vi "CCD Exposure Time Control.vi"(8 "error in (no error)":errorcluster, 11 "CCD in":refnum<class "CCD.lvclass">) -> (0 "error out":errorcluster, 3 "CCD out":refnum<class "CCD.lvclass">)   [LabVIEW 2020, in "Examples.lvlib"]
doc: "Example on how to use the timer resolution to to achieve a exposure time in mili seconds."
uses:
  Examples.lvlib
  Classes/CCD/CCD.lvclass
panel:
  out "time [ms] or [us]":i32
  out "resolutionToken":i32
  # "See Block Diagram\nfor explanation"
  # "Connector Pane"
  # "Locals"
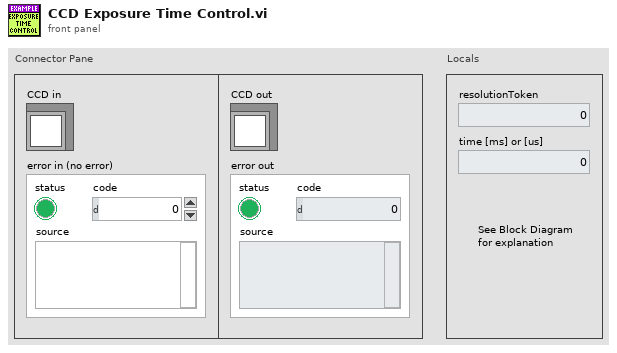
[diagram p1: front panel]
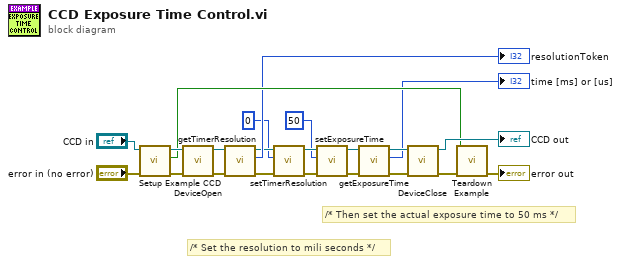
[diagram p0: block diagram]
diagram:
  # "/* Then set the actual exposure time to 50 ms */"
  # "/* Set the resolution to mili seconds */"
  n1 = call "Setup Example CCD.vi"("error in (no error)"="error in (no error)", "CCD in"="CCD in") -> ("error out"=w21:errorcluster, "Module Was Already Running?"=w15:bool, "CCD out"=w17:refnum<class "CCD.lvclass">)  [unwired: 7 in]
  n2 = call-dynamic "DeviceOpen.vi"("error in (no error)"=w21, "CCD in"=w17) -> ("error out"=w13:errorcluster, "CCD out"=w14:refnum<class "CCD.lvclass">)  [unwired: 6 in, 2 out]
  n3 = call "getTimerResolution.vi"("error in (no error)"=w13, "CCD in"=w14) -> ("error out"=w10:errorcluster, "resolutionToken"=→"resolutionToken":i32, "CCD out"=w11:refnum<class "CCD.lvclass">)  [unwired: 7 in]
  n4 = call "setTimerResolution.vi"("error in (no error)"=w10, "resolutionToken"=0, "CCD in"=w11) -> ("error out"=w7:errorcluster, "CCD out"=w8:refnum<class "CCD.lvclass">)  [unwired: 5 in, 2 out]
  n5 = call "setExposureTime.vi"("error in (no error)"=w7, "exposure time [ms] or [us]"=50, "CCD in"=w8) -> ("error out"=w6:errorcluster, "CCD out"=w3:refnum<class "CCD.lvclass">)  [unwired: 5 in, 2 out]
  n6 = call "getExposureTime.vi"("error in (no error)"=w6, "CCD in"=w3) -> ("error out"=w4:errorcluster, "time [ms] or [us]"=→"time [ms] or [us]":i32, "CCD out"=w2:refnum<class "CCD.lvclass">)  [unwired: 7 in]
  n7 = call-dynamic "DeviceClose.vi"("error in (no error)"=w4, "CCD in"=w2) -> ("error out"=w18:errorcluster, "CCD out"=→"CCD out":refnum<class "CCD.lvclass">)  [unwired: 5 in, 3 out]
  n8 = call "Teardown Example.vi"("error in (no error)"=w18, "Module Was Already Running?"=w15) -> ("error out"=→"error out":errorcluster)  [unwired: 9 in]
